vi "Control_WaterPump.vi"(2 "Pump 1 Signal":bool, 3 "Pump 2 Signal":bool) -> (0 "Pump 1 check":bool, 1 "Pump 2 check":bool)   [LabVIEW 2022 SP3]
uses:
  <vilib>/DAQmx/write.llb/DAQmx Write (Digital Bool 1Line 1Point).vi
  <vilib>/DAQmx/create/channels.llb/DAQmx Create Channel (DO-Digital Output).vi
panel:
  in  "stop 2":bool
  in  "Pump 2":tag
  in  "stop":bool
  in  "Pump 1":tag
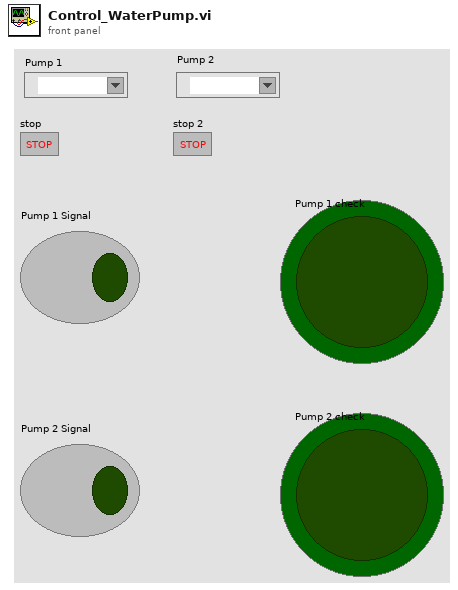
[diagram p1: front panel]
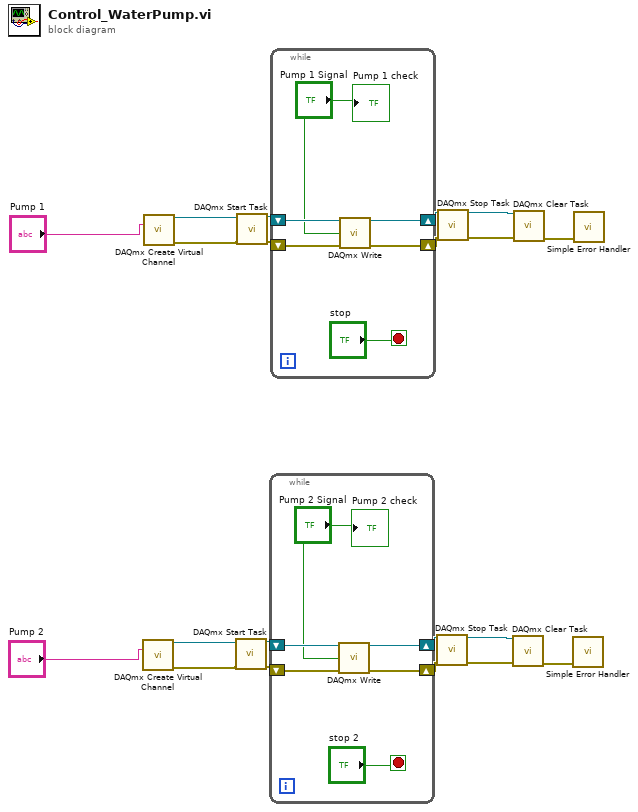
[diagram p0: block diagram]
diagram:
  n1 = call-poly <vilib>:"DAQmx Create Virtual Channel.vi"("lines"="Pump 2") -> ("task out"=w9:refnum<k21>, "error out"=w8:errorcluster)  [unwired: 13 in]
  n2 = call-poly <vilib>:"DAQmx Create Virtual Channel.vi"("lines"="Pump 1") -> ("task out"=w19:refnum<k21>, "error out"=w18:errorcluster)  [unwired: 13 in]
  n3 = call <vilib>:"DAQmx Start Task.vi"("task/channels in"=w9, "error in"=w8) -> ("task out"=w4:refnum<k21>, "error out"=w1:errorcluster)  [unwired: 12 in]
  n4 = call <vilib>:"DAQmx Start Task.vi"("task/channels in"=w19, "error in"=w18) -> ("task out"=w14:refnum<k21>, "error out"=w11:errorcluster)  [unwired: 12 in]
  n5 = while {
    shift-right: [w25] -> w3
    shift-left: w4 -> [w26]
    shift-right: [w24] -> w2
    shift-left: w1 -> [w23]
    stop <- "stop 2" stop-if-true
    n6 = call-poly <vilib>:"DAQmx Write.vi"("task/channels in"=w26, "data"="Pump 2 Signal", "error in"=w23) -> ("task out"=w25:refnum<k21>, "error out"=w24:errorcluster)  [unwired: 10 in, 1 out]
    "Pump 2 check" <- "Pump 2 Signal"
  }
  n7 = while {
    shift-right: [w31] -> w13
    shift-left: w14 -> [w32]
    shift-right: [w30] -> w12
    shift-left: w11 -> [w29]
    stop <- "stop" stop-if-true
    n8 = call-poly <vilib>:"DAQmx Write.vi"("task/channels in"=w32, "data"="Pump 1 Signal", "error in"=w29) -> ("task out"=w31:refnum<k21>, "error out"=w30:errorcluster)  [unwired: 10 in, 1 out]
    "Pump 1 check" <- "Pump 1 Signal"
  }
  n9 = call <vilib>:"DAQmx Stop Task.vi"("task/channels in"=w3, "error in"=w2) -> ("task out"=w7:refnum<k21>, "error out"=w6:errorcluster)  [unwired: 12 in]
  n10 = call <vilib>:"DAQmx Stop Task.vi"("task/channels in"=w13, "error in"=w12) -> ("task out"=w17:refnum<k21>, "error out"=w16:errorcluster)  [unwired: 12 in]
  n11 = call <vilib>:"DAQmx Clear Task.vi"("task in"=w7, "error in"=w6) -> ("error out"=w5:errorcluster)  [unwired: 13 in]
  n12 = call <vilib>:"DAQmx Clear Task.vi"("task in"=w17, "error in"=w16) -> ("error out"=w15:errorcluster)  [unwired: 13 in]
  n13 = call <vilib>:"Simple Error Handler.vi"("error in (no error)"=w5) -> ()  [unwired: 4 in, 5 out]
  n14 = call <vilib>:"Simple Error Handler.vi"("error in (no error)"=w15) -> ()  [unwired: 4 in, 5 out]
